vi "Actor Core.vi"(8 "error in":errorcluster, 11 "CS++Nanotec in":refnum<class "CS++Nanotec.lvclass">) -> (0 "error out":errorcluster, 3 "Actor out":refnum<class "Actor.lvclass">)   [LabVIEW 2015, in "CS++Nanotec.lvlib" / "CS++Nanotec.lvclass"]
doc: "(<B>Filename</B>: Actor Framework.lvlib:Actor.lvclass:Actor Core.vi)\n\nReceives messages to the actor, reacts to them, and initiates any error handling that may shut the actor down.\n\nDescendant classes may override this VI to append parallel tasks for the actor to complete while it handles messages. Overrides use the Call Parent Method node."
uses:
  CS++Nanotec.lvclass
  <vilib>/ActorFramework/Actor/Actor.lvclass
  CSPP_Core/Actors/CS++BaseActor/CS++BaseActor.lvclass/CS++BaseActor.ctl
  CS++Nanotec.lvclass/CS++Nanotec.ctl
  CSPP_Core/Classes/CS++ProcessVariables/ProcessVariable/PV.lvclass
  CSPP_Core/Classes/CS++ProcessVariables/ProcessVariable/PV.lvclass/PV.ctl
  <vilib>/ActorFramework/Message Enqueuer/Message Priority.ctl
  <vilib>/ActorFramework/Actor/Actor.lvclass/Actor.ctl
  <vilib>/ActorFramework/Message Enqueuer/Message Enqueuer.lvclass/Message Enqueuer.ctl
  <vilib>/ActorFramework/Report Error Msg/Report Error Msg.lvclass/Report Error Msg.ctl
  CSPP_Core/Classes/CS++ProcessVariables/ProcessVariable/Write Data.vi
  CSPP_Core/Classes/CS++ProcessVariables/ProcessVariable/Write Timestamp.vi
  <vilib>/ActorFramework/Message Enqueuer/Init from Existing Queue.vi
  <vilib>/ActorFramework/Message Enqueuer/Enqueue.vi
  <vilib>/ActorFramework/Message Priority Queue/Priority Enqueue.vi
  CSPP_DeviceBase/CS++Motor/CS++Motor.lvclass
  <vilib>/ActorFramework/Message Enqueuer/Message Enqueuer.lvclass
  <vilib>/ActorFramework/Report Error Msg/Report Error Msg.lvclass
  CSPP_Core/Actors/CS++BaseActor/CS++BaseActor.lvclass
  instr.lib/NanotecSMCPD/NanotecSMCPDDriver.lvlib
  CSPP_Core/Classes/CS++ProcessVariables/PVConnection/PVConnection.lvclass
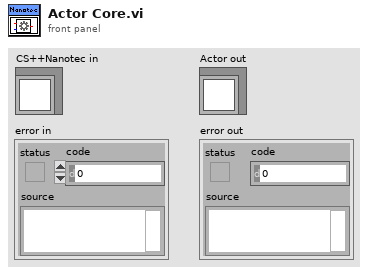
[diagram p1: front panel]
types:
  T1 = typedef "Actor Framework.lvlib/Message Enqueuer.lvclass/Message Priority.ctl" = enum16{"Low", "Normal", "High"}
  T2 = cluster{"Stop Event":refnum<user-event>, "Pos Update Event":refnum<user-event>, "Reset Event":refnum<user-event>}
  T3 = typedef "NanotecSMCPDDriver.lvlib/NanotecSMCPDDriver.status type.ctl" = cluster{"ready":bool, "homePosition":bool, "positionError":bool, "input1":bool, "controllerMode":enum16{"unknown", "position", "speed", "flagPosition", "clockDirection", "analog", "joystick", "unused"}, "unused":bool}
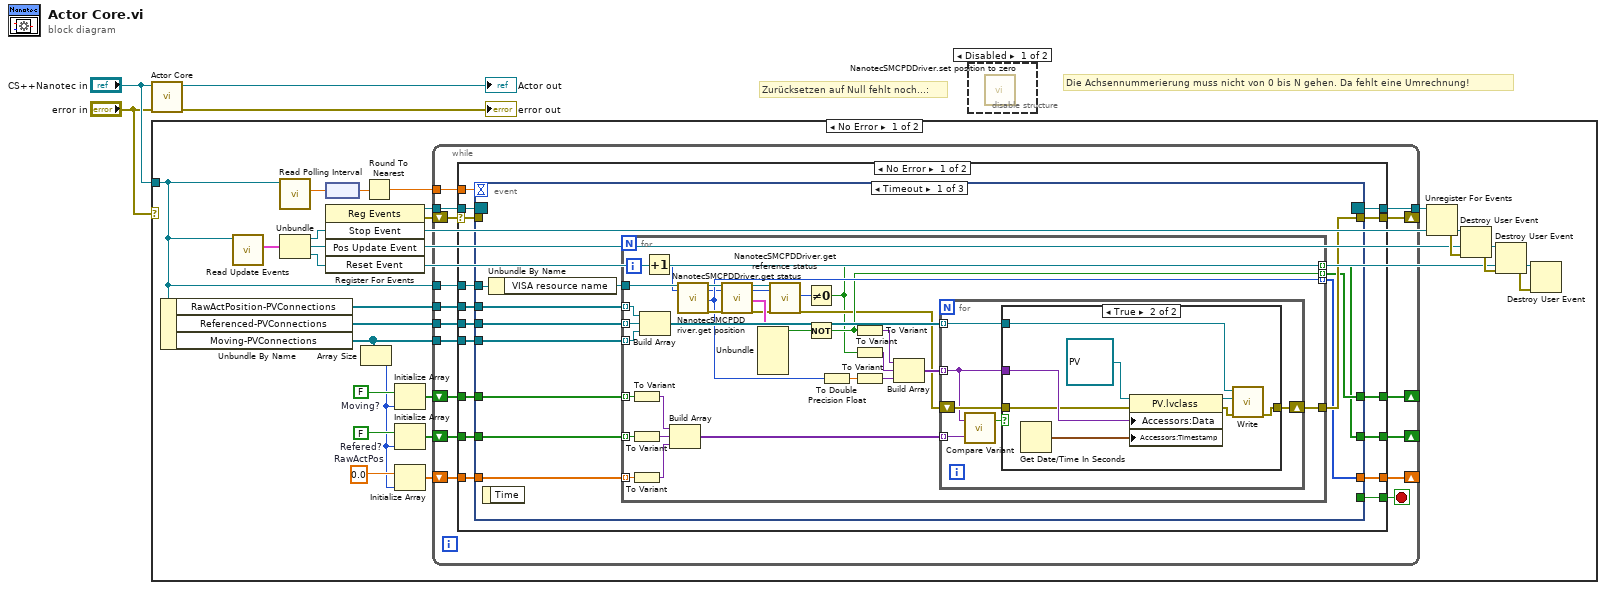
[diagram p0: block diagram]
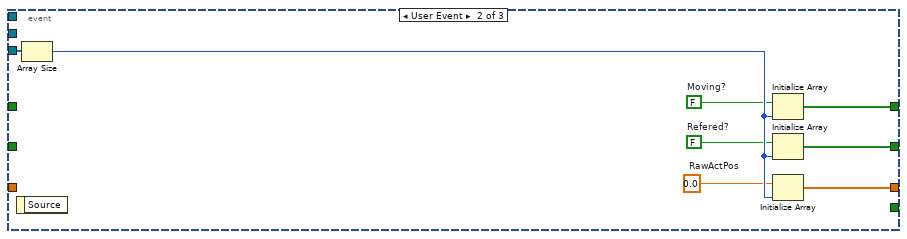
[diagram p4: hidden frame]
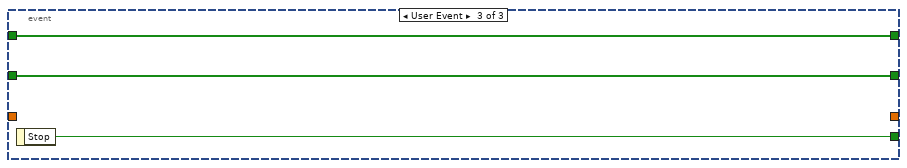
[diagram p5: hidden frame]
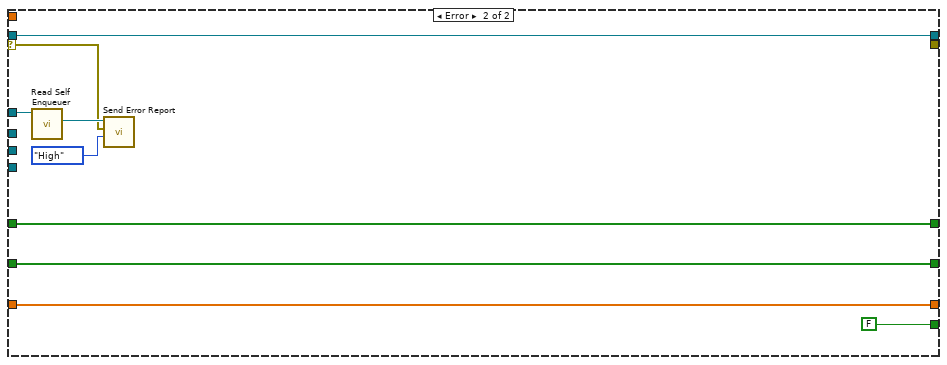
[diagram p6: hidden frame]
diagram:
  # "Die Achsennummerierung muss nicht von 0 bis N gehen. Da fehlt eine Umrechnung!"
  # "Zurücksetzen auf Null fehlt noch...:"
  n1 = call-parent "Actor Core.vi"("error in"="error in", "CS++Motor in"="CS++Nanotec in") -> ("error out"=→"error out":errorcluster, "Actor out"=→"Actor out":refnum<class "Actor.lvclass">)  [unwired: 8 in]
  n2 = case shown="No Error" "error in" {
    tunnel: "CS++Nanotec in" -> [w15 _]
    frame No Error {
      w8 = 0.0  # RawActPos
      w12 = FALSE  # Refered?
      w13 = FALSE  # Moving?
      n3 = Unbundle By Name(w15) -> ("RawActPosition-PVConnections"=w14:refnum<class "PVConnection.lvclass">[], "Referenced-PVConnections"=w16:refnum<class "PVConnection.lvclass">[], "Moving-PVConnections"=w11:refnum<class "PVConnection.lvclass">[])
      n4 = call "Read Update Events.vi"("CS++Nanotec in"=w15) -> ("Update Events"=w26:T2)  [unwired: 8 in, 2 out]
      n5 = call "Read Polling Interval.vi"("CS++BaseActor in"=w15) -> ("Polling Interval"=w27:dbl[unit])  [unwired: 8 in, 2 out]
      n6 = Unbundle(w26) -> ("Stop Event"=w22:refnum<user-event>, "Pos Update Event"=w19:refnum<user-event>, "Reset Event"=w18:refnum<user-event>)
      n7 = node(w27) -> (w28:dbl)
      n8 = register-events(w22, w19, w18) -> (reference out=w24:refnum<event-registration>, error out=w5:errorcluster)  [unwired: 2 in]
      n9 = Array Size(array=w11) -> (size(s)=w7:i32)
      n10 = Round To Nearest(number=w28) -> (nearest integer value=w25:dbl)
      n11 = Initialize Array(w13, w7) -> (w10:bool[])
      n12 = Initialize Array(w12, w7) -> (w9:bool[])
      n13 = Initialize Array(w8, w7) -> (w6:dbl[])
      n14 = while {
        tunnel: w25 -> [w44]
        tunnel: w24 -> [w43]
        tunnel: [w42] -> w23
        tunnel: w11 -> [w40]
        tunnel: w16 -> [w39]
        tunnel: w14 -> [w38]
        tunnel: w15 -> [w37]
        shift-right: [w33] -> _
        shift-left: w9 -> [w35]
        shift-right: [w34] -> _
        shift-left: w10 -> [w36]
        shift-right: [w31] -> _
        shift-left: w6 -> [w32]
        shift-right: [w29] -> _
        shift-left: w5 -> [w30]
        stop <- w41 stop-if-true
        n15 = case shown="No Error" w30 {
          selector: w30 -> [w46 w137]
          tunnel: w44 -> [w60 _]
          tunnel: w43 -> [w59 w140]
          tunnel: [w58 w140] -> w42
          tunnel: [w57 FALSE ("Stop")] -> w41
          tunnel: w40 -> [w56 _]
          tunnel: w39 -> [w55 _]
          tunnel: w38 -> [w54 _]
          tunnel: w37 -> [w53 w135]
          tunnel: w36 -> [w52 w134]
          tunnel: w35 -> [w51 w133]
          tunnel: [w50 w134] -> w34
          tunnel: [w49 w133] -> w33
          tunnel: w32 -> [w48 w132]
          tunnel: [w47 w132] -> w31
          tunnel: [w45 _] -> w29
          frame No Error {
            n16 = event shown="[0] Timeout" {
              selector: w59 -> [_ _ _]
              dyn-events: [_ _ _] -> w58
              timeout: w60 -> [_ _ _]
              tunnel: [_ _ w131] -> w57
              tunnel: w56 -> [w65 w121 _]
              tunnel: w55 -> [w66 _ _]
              tunnel: w54 -> [w67 _ _]
              tunnel: w53 -> [w72 _ _]
              tunnel: w52 -> [w69 _ w130]
              tunnel: w51 -> [w68 _ w129]
              tunnel: [w62 w124 w130] -> w50
              tunnel: [w61 w123 w129] -> w49
              tunnel: [w70 _ _] -> w45
              tunnel: w48 -> [w64 _ _]
              tunnel: [w63 w122 _] -> w47
              tunnel: w46 -> [_ _ _]
              event Timeout {
                n17 = event-data() -> ()  [unwired: 1 in, 1 out]
                n18 = Unbundle By Name(w72) -> ("VISA resource name"=w71:refnum<visa-resource-name>)
                n19 = for {
                  tunnel: w71 -> [w105]
                  tunnel: [w83] -> w70
                  tunnel: w69 -> [w96] mode=indexing
                  tunnel: w68 -> [w95] mode=indexing
                  tunnel: w67 -> [w100] mode=indexing
                  tunnel: w66 -> [w99] mode=indexing
                  tunnel: w65 -> [w98] mode=indexing
                  tunnel: w64 -> [w94] mode=indexing
                  tunnel: [w82] -> w63 mode=indexing
                  tunnel: [w81] -> w62 mode=indexing
                  tunnel: [w73] -> w61 mode=indexing
                  i -> [w102]
                  n20 = To Variant(anything=w96) -> (Variant=w93:variant)
                  n21 = To Variant(anything=w95) -> (Variant=w92:variant)
                  n22 = To Variant(anything=w94) -> (Variant=w91:variant)
                  n23 = Build Array(w100, w99, w98) -> (w97:refnum<class "PVConnection.lvclass">[])
                  n24 = Increment(x=w102) -> (x+1=w101:i32)
                  n25 = Build Array(w93, w92, w91) -> (w84:variant[])
                  n26 = call "NanotecSMCPDDriver.get position.vi"("VISA resource name"=w105, "contollerID"=w101) -> ("VISA resource name out"=w104:refnum<visa-resource-name>, "contollerID out"=w77:i32, "actPosition [usteps]"=w82:i32, "error out"=w103:errorcluster)  [unwired: 14 in]
                  n27 = call "NanotecSMCPDDriver.get status.vi"("VISA resource name"=w104, "contollerID"=w77, "error in (no error)"=w103) -> ("VISA resource name out"=w79:refnum<visa-resource-name>, "contollerID out"=w76:i32, "actStatus"=w90:T3, "error out"=w78:errorcluster)  [unwired: 13 in]
                  n28 = Unbundle(w90) -> ("ready"=w88:bool)  [unwired: 5 out]
                  n29 = call "NanotecSMCPDDriver.get reference status.vi"("VISA resource name"=w79, "contollerID"=w76, "error in (no error)"=w78) -> ("referenced"=w74:u8, "error out"=w75:errorcluster)  [unwired: 13 in, 2 out]
                  n30 = Not Equal To 0?(x=w74) -> (x != 0?=w73:bool)
                  n31 = Not(x=w88) -> (.not. x?=w81:bool)
                  n32 = To Double Precision Float(number=w82) -> (double precision float=w80:dbl)
                  n33 = To Variant(anything=w81) -> (Variant=w87:variant)
                  n34 = To Variant(anything=w73) -> (Variant=w86:variant)
                  n35 = To Variant(anything=w80) -> (Variant=w89:variant)
                  n36 = Build Array(w87, w86, w89) -> (w85:variant[])
                  n37 = for {
                    tunnel: w97 -> [w111] mode=indexing
                    tunnel: w85 -> [w107] mode=indexing
                    tunnel: w84 -> [w108] mode=indexing
                    shift-right: [w109] -> w83
                    shift-left: w75 -> [w110]
                    n38 = call "Compare Variant.vi"("Variant 2"=w108, "Variant 1"=w107) -> ("Equal?"=w106:bool)  [unwired: 1 out]
                    n39 = case shown="True" w106 {
                      tunnel: w111 -> [_ w116]
                      tunnel: w107 -> [_ w115]
                      tunnel: w110 -> [w112 w114]
                      tunnel: [w112 w113] -> w109
                      frame False {
                      }
                      frame True {
                        n40 = Get Date/Time In Seconds() -> (seconds since 1Jan1904=w118:timestamp)
                        n41 = property class="PV.lvclass"(reference=refnum<class "PV.lvclass"> refnum ("PV"), error in=w114, "Accessors:Data"=w115, "Accessors:Timestamp"=w118) -> (reference out=w120:refnum<class "PV.lvclass">, error out=w119:errorcluster)
                        n42 = call "Write.vi"("error in (no error)"=w119, "PV"=w120, "PVConnection in"=w116) -> ("error out"=w113:errorcluster)  [unwired: 7 in, 1 out]
                      }
                    }
                  }
                }
              }
              event User Event {
                w127 = 0.0  # RawActPos
                w126 = FALSE  # Refered?
                w125 = FALSE  # Moving?
                n43 = event-data() -> ()  [unwired: 1 in, 1 out]
                n44 = Array Size(array=w121) -> (size(s)=w128:i32)
                n45 = Initialize Array(w125, w128) -> (w124:bool[])
                n46 = Initialize Array(w126, w128) -> (w123:bool[])
                n47 = Initialize Array(w127, w128) -> (w122:dbl[])
              }
              event User Event {
                n48 = event-data() -> ("Stop"=w131:bool)  [unwired: 1 in]
              }
            }
          }
          frame Error {
            n49 = call <vilib>:"Read Self Enqueuer.vi"("Actor"=w135) -> ("Self Enqueuer"=w139:refnum<class "Message Enqueuer.lvclass">)  [unwired: 10 in]
            n50 = call <vilib>:"Send Error Report.vi"("Message Priority (Normal)"=Message_Priority."High", "Error From Sender"=w137, "Message Enqueuer"=w139) -> ()  [unwired: 8 in, 1 out]
          }
        }
      }
      n51 = Unregister For Events(event registration refnum=w23) -> (error out=w21:errorcluster)  [unwired: 1 in]
      n52 = Destroy User Event(user event=w22, error in=w21) -> (error out=w20:errorcluster)
      n53 = Destroy User Event(user event=w19, error in=w20) -> (error out=w17:errorcluster)
      n54 = Destroy User Event(user event=w18, error in=w17) -> ()  [unwired: 1 out]
    }
    frame Error {
    }
  }
  n55 = disable-structure shown="Disabled" {
    frame Disabled {
      n56 = call "NanotecSMCPDDriver.set position to zero.vi"() -> ()  [unwired: 17 in, 3 out]
    }
    frame Enabled {
    }
  }
